vi "Strip Class Function Name.vi"(4 "Strip vi extension(T)":bool=TRUE, 5 "File Full Path Name":string="libpname.lvlibp:libname.lvlib:classname.lvclass:funcname.vi") -> (0 "library name":string, 1 "Class name":string, 2 "Function Name":string="replace memory subs")   [LabVIEW 2017]
doc: "Splits a VI's full path into the library name, the class name and the function name. Set Strip vi extension(T) to remove the .vi extension from the function name."
uses:
  82d5ef48-2c95-4ac8-8452-541d4ca00c93.vi
  8c0b350f-6b41-4dd8-8255-dad520baa4a5.vi
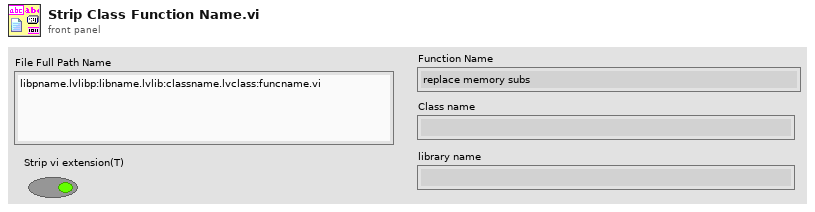
[diagram p1: front panel]
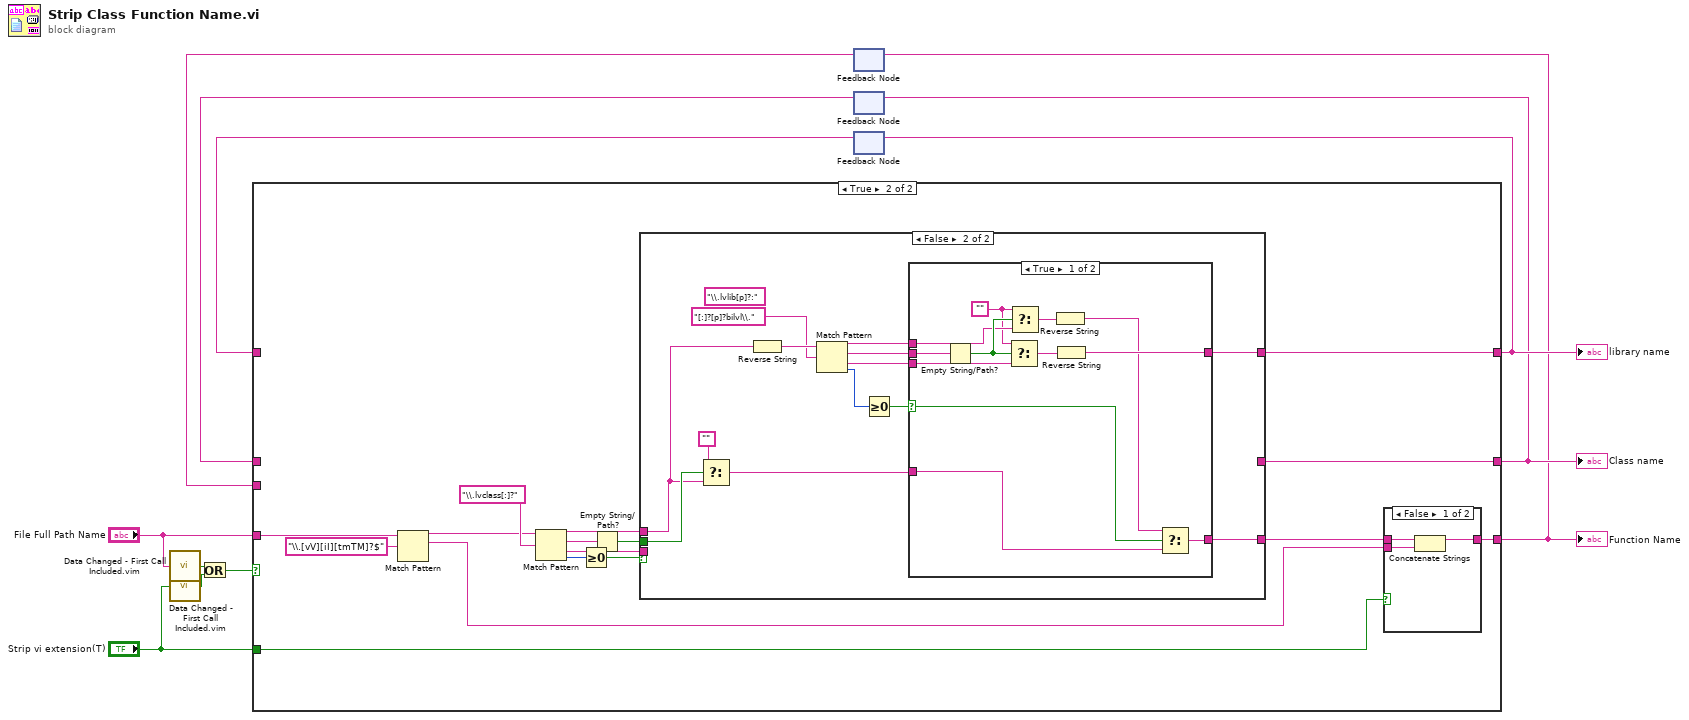
[diagram p0: block diagram]
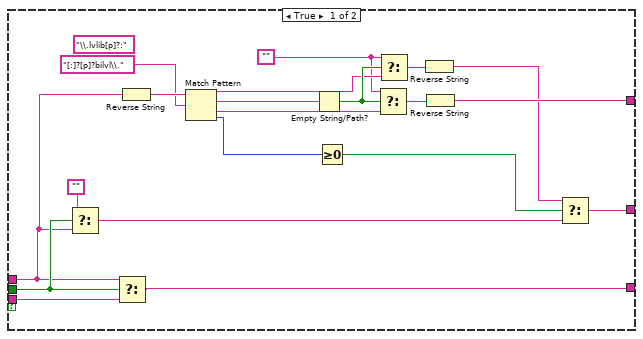
[diagram p3: hidden frame]
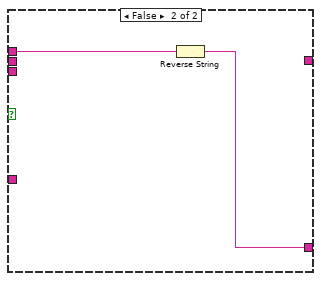
[diagram p4: hidden frame]
diagram:
  n1 = call "Data Changed - First Call Included.vim"("Variant"="File Full Path Name") -> ("Changed"=w9:bool)
  n2 = call "Data Changed - First Call Included.vim"("Variant"="Strip vi extension(T)") -> ("Changed"=w8:bool)
  n3 = Or(x=w9, y=w8) -> (x .or. y?=w7:bool)
  n4 = feedback #1() -> (w1:string)  [unwired: 1 in]
  n5 = feedback #2() -> (w2:string)  [unwired: 1 in]
  n6 = feedback #3() -> (w3:string)  [unwired: 1 in]
  n7 = case shown="True" w7 {
    tunnel: [w12 w27] -> w4
    tunnel: [w14 w24] -> w6
    tunnel: [w13 w23] -> w5
    tunnel: "File Full Path Name" -> [_ w16]
    tunnel: "Strip vi extension(T)" -> [_ w15]
    tunnel: w3 -> [w14 _]
    tunnel: w2 -> [w13 _]
    tunnel: w1 -> [w12 _]
    frame False {
    }
    frame True {
      n8 = Match Pattern(string=w16, regular expression="\\.[vV][iI][tmTM]?$") -> (before substring=w25:string, match substring=w17:string)  [unwired: 1 in, 2 out]
      n9 = Match Pattern(string=w25, regular expression="\\.lvclass[:]?") -> (before substring=w22:string, match substring=w19:string, after substring=w30:string, offset past match=w21:i32)  [unwired: 1 in]
      n10 = Greater Or Equal To 0?(x=w21) -> (x >= 0?=w20:bool)
      n11 = Empty String/Path?(string/path=w19) -> (empty?=w18:bool)
      n12 = case shown="False" w20 {
        tunnel: w30 -> [w50 _]
        tunnel: [w49 w51] -> w26
        tunnel: w18 -> [w48 w63]
        tunnel: [w45 w60] -> w24
        tunnel: [w33 _] -> w23
        tunnel: w22 -> [w31 w52]
        frame True {
          w32 = ""
          (unwired) "\\.lvlib[p]?:" ("regular expression")
          n13 = Select(t="", s=w48, f=w31) -> (s? t:f=w34:string)
          n14 = Select(t=w31, s=w48, f=w50) -> (s? t:f=w49:string)
          n15 = Reverse String(1:w31) -> (0:w46:string)
          n16 = Match Pattern(string=w46, regular expression="[:]?[p]?bilvl\\.") -> (before substring=w39:string, match substring=w44:string, after substring=w43:string, offset past match=w37:i32)  [unwired: 1 in]
          n17 = Empty String/Path?(string/path=w44) -> (empty?=w41:bool)
          n18 = Greater Or Equal To 0?(x=w37) -> (x >= 0?=w36:bool)
          n19 = Select(t=w32, s=w41, f=w43) -> (s? t:f=w42:string)
          n20 = Select(t=w32, s=w41, f=w39) -> (s? t:f=w40:string)
          n21 = Reverse String(1:w40) -> (0:w35:string)
          n22 = Reverse String(1:w42) -> (0:w45:string)
          n23 = Select(t=w35, s=w36, f=w34) -> (s? t:f=w33:string)
        }
        frame False {
          (unwired) "\\.lvlib[p]?:" ("regular expression")
          n24 = Select(t="", s=w63, f=w52) -> (s? t:f=w53:string)
          n25 = Reverse String(1:w52) -> (0:w61:string)
          n26 = Match Pattern(string=w61, regular expression="[:]?[p]?bilvl\\.") -> (before substring=w57:string, match substring=w59:string, after substring=w58:string, offset past match=w55:i32)  [unwired: 1 in]
          n27 = Greater Or Equal To 0?(x=w55) -> (x >= 0?=w54:bool)
          n28 = case shown="True" w54 {
            selector: w54 -> [w68 _]
            tunnel: [w75 _] -> w60
            tunnel: w59 -> [w74 _]
            tunnel: w58 -> [w73 _]
            tunnel: w57 -> [w69 w76]
            tunnel: w53 -> [w66 _]
            tunnel: [w64 w77] -> w51
            frame True {
              w65 = ""
              n29 = Empty String/Path?(string/path=w74) -> (empty?=w71:bool)
              n30 = Select(t=w65, s=w71, f=w73) -> (s? t:f=w72:string)
              n31 = Select(t=w65, s=w71, f=w69) -> (s? t:f=w70:string)
              n32 = Reverse String(1:w70) -> (0:w67:string)
              n33 = Reverse String(1:w72) -> (0:w75:string)
              n34 = Select(t=w67, s=w68, f=w66) -> (s? t:f=w64:string)
            }
            frame False {
              n35 = Reverse String(1:w76) -> (0:w77:string)
            }
          }
        }
      }
      n36 = case shown="False" w15 {
        tunnel: w26 -> [w80 w81]
        tunnel: [w79 w81] -> w27
        tunnel: w17 -> [w78 _]
        frame False {
          n37 = Concatenate Strings(w80, w78) -> (w79:string)
        }
        frame True {
        }
      }
    }
  }
  "Function Name" <- w4
  "library name" <- w6
  "Class name" <- w5
  n38 = feedback-in #1(w4) -> ()
  n39 = feedback-in #2(w5) -> ()
  n40 = feedback-in #3(w6) -> ()
